vi "IR Sensor.vi"(11 "Enum":enum16{"Init", "Run", "End"}(ring)) -> ()   [LabVIEW 2011]
uses:
  TypeDefs/Digital Module 1.ctl
  <vilib>/Rock Robotics/SystemInterfaces/Typedef/FPGA_TypedefDigitalModule.ctl
  <vilib>/Rock Robotics/SystemInterfaces/DIO/FPGA_DIOChannel.ctl
panel:
  out "Bottom Front":bool
  in  "Digital Module A":T1={"Module"=enum."Digital Module 1", "Left Enc A"=enum."DIO 1", "Left Enc B"=enum."DIO 2", "Right Enc A"=enum."DIO 3", "Right Enc B"=enum."DIO 4", "Grab Ball"=enum."DIO 5", "Ball Input"=enum."DIO 6", "Ball Output"=enum."DIO 7", "Shooter Tachometer"=enum."DIO 8", "Auto Switch 1"=enum."DIO 9", "Auto Switch 2"=enum."DIO 10", "Auto Switch 3"=enum."DIO 11", "Arm Upper Limit"=enum."DIO 12", "Arm Lower Limit"=enum."DIO 13", "Robot 1/2 Switch"=enum."DIO 14"}
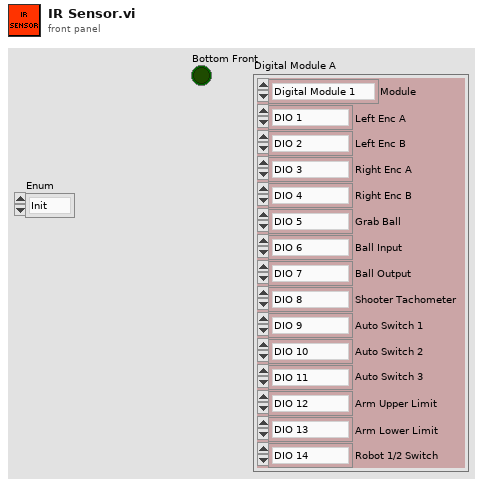
[diagram p1: front panel]
types:
  T1 = typedef "Digital Module 1.ctl" = cluster{"Module":T2, "Left Enc A":T3, "Left Enc B":T3, "Right Enc A":T3, "Right Enc B":T3, "Grab Ball":T3, "Ball Input":T3, "Ball Output":T3, "Shooter Tachometer":T3, "Auto Switch 1":T3, "Auto Switch 2":T3, "Auto Switch 3":T3, "Arm Upper Limit":T3, "Arm Lower Limit":T3, "Robot 1/2 Switch":T3}
  T2 = typedef "FPGA_TypedefDigitalModule.ctl" = enum16{"Digital Module 1", "Digital Module 2"}
  T3 = typedef "FPGA_DIOChannel.ctl" = enum8{"DIO 1", "DIO 2", "DIO 3", "DIO 4", "DIO 5", "DIO 6", "DIO 7", "DIO 8", "DIO 9", "DIO 10", "DIO 11", "DIO 12", "DIO 13", "DIO 14", "Invalid"}
  T4 = typedef "WPI_DigitalInputDevRef.ctl" = cluster{"DevStatus":errorcluster, "DIO Channel":T3, "Digital Module":T2}
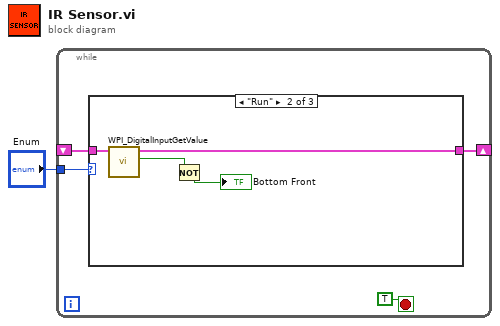
[diagram p0: block diagram]
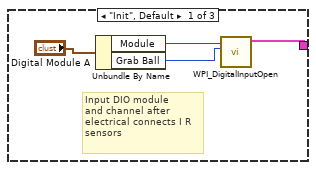
[diagram p2: hidden frame]
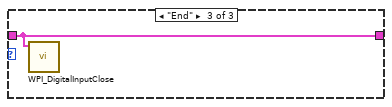
[diagram p3: hidden frame]
diagram:
  n1 = while {
    tunnel: "Enum" -> [w4]
    shift-right: [w3] -> _
    shift-left: _ -> [w2]
    stop <- TRUE stop-if-true
    n2 = case shown="\"Run\"" w4 {
      tunnel: [w9 w12 w14] -> w3
      tunnel: w2 -> [_ w13 w14]
      frame "Init", Default {
        # "Input DIO module \nand channel after \nelectrical connects I R \nsensors"
        n3 = Unbundle By Name("Digital Module A") -> ("Module"=w7:T2, "Grab Ball"=w6:T3)
        n4 = call <vilib>:"WPI_DigitalInputOpen.vi"("DIO Channel"=w6, "Digital Module (Module 1)"=w7) -> ("DigitalInputDevRef"=w9:T4)  [unwired: 1 in, 8 out]
      }
      frame "Run" {
        n5 = call <vilib>:"WPI_DigitalInputGetValue.vi"("DigitalInputDevRef"=w13) -> ("Value"=w11:bool, "DigitalInputDevRef"=w12:T4)  [unwired: 1 in, 8 out]
        n6 = Not(x=w11) -> (.not. x?=→"Bottom Front":bool)
      }
      frame "End" {
        n7 = call <vilib>:"WPI_DigitalInputClose.vi"("DigitalInputDevRef"=w14) -> ()  [unwired: 1 in, 10 out]
      }
    }
  }
